vi "Set Data Ready Event.vi"(8 "error in (no error)":errorcluster, 11 "dataevent":u32) -> (0 "error out":errorcluster, 3 "dataevent out":u32)   [LabVIEW 2023, in "vmmsolib.lvlib"]
doc: "DLL_API void WINAPI SetDataReadyEvent(HANDLE dataevent);"
uses:
  vmmsolib.lvlib
  vmmso.dll
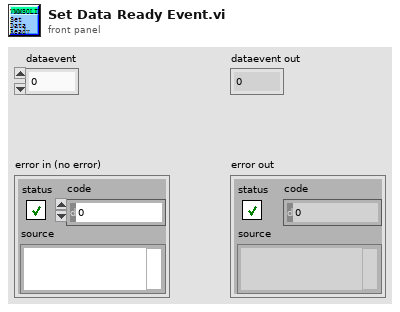
[diagram p1: front panel]
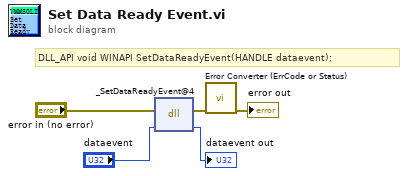
[diagram p0: block diagram]
diagram:
  # "DLL_API void WINAPI SetDataReadyEvent(HANDLE dataevent);"
  n1 = dll-call lib="D:/VmMsoSDK/demo-Labview/2023/vmmsolib/vmmso.*" fn="_SetDataReadyEvent@4"(error in="error in (no error)", "dataevent"="dataevent") -> (error out=w2:errorcluster, "dataevent"=→"dataevent out":u32)  [unwired: 3 in, 1 out]
  n2 = call "Error Converter (ErrCode or Status).vi"("error in (no error)"=w2) -> ("error out"=→"error out":errorcluster)  [unwired: 10 in]
